vi "Corners to Rectangle Tim's version.vi"(10 "Rectangle Descriptor":T1) -> (2 "output cluster":T3={"diameter points"={"first point"={"x"=0.0, "y"=0.0}, "projected point"={"x"=0.0, "y"=0.0}}, "normalized center"={"x"=0.0, "y"=0.0}, "Overall Score"=0.0, "Distance (ft)"=0.0, "Offset Angle"=0.0, "Tag corner points"=[], "Tag Center"={"X"=0.0, "Y"=0.0}, "Tag Yaw"=0.0, "Tag Pitch"=0.0, "Target Roll (deg)"=0.0, "AprilTag Number"=68} {"Tag Center"."Y" format="%0.2f"; "Tag Center"."X" format="%0.2f"})   [LabVIEW 2023]
uses:
  AprilTag Target Fields.ctl
panel:
  in  "tag info":T2={"tag ID"=0, "Center"={"X"=0.0, "Y"=0.0}, "homography matrix"=[], "decision margin"=0.0, "Hamming Dist"=0, "corner points"=[], "Tag Family"="36h11"}
  # "Bottom Left"
  # "Bottom Right"
  # "Top Right"
  # "Top Left"
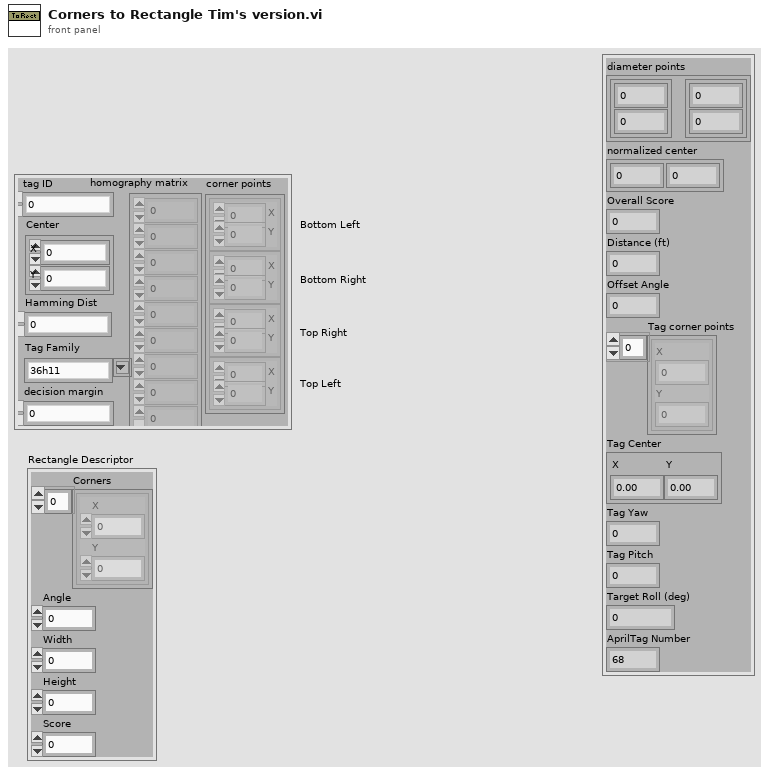
[diagram p1: front panel]
types:
  T1 = cluster{"Corners":cluster{"X":sgl, "Y":sgl}[], "Angle":dbl, "Width":dbl, "Height":dbl, "Score":dbl}
  T2 = cluster{"tag ID":i32, "Center":cluster{"X":dbl, "Y":dbl}, "homography matrix":dbl[], "decision margin":dbl, "Hamming Dist":i32, "corner points":cluster{"X":dbl, "Y":dbl}[], "Tag Family":string}
  T3 = typedef "AprilTag Target Fields.ctl" = cluster{"diameter points":cluster{"first point":cluster{"x":dbl, "y":dbl}, "projected point":cluster{"x":dbl, "y":dbl}}, "normalized center":cluster{"x":dbl, "y":dbl}, "Overall Score":dbl, "Distance (ft)":dbl, "Offset Angle":dbl, "Tag corner points":cluster{"X":dbl, "Y":dbl}[], "Tag Center":cluster{"X":dbl, "Y":dbl}, "Tag Yaw":dbl, "Tag Pitch":dbl, "Target Roll (deg)":dbl, "AprilTag Number":i32}
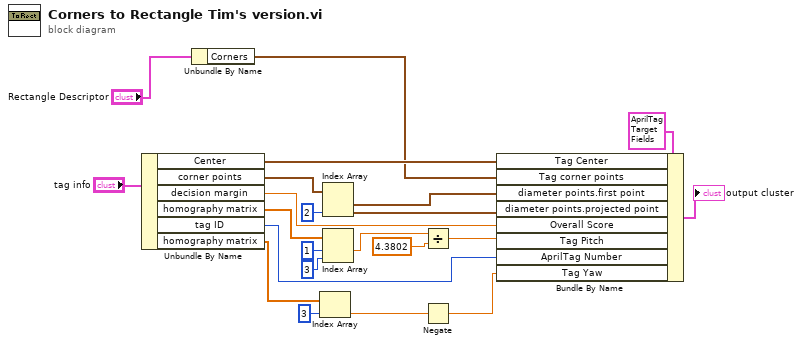
[diagram p0: block diagram]
diagram:
  n1 = Unbundle By Name("tag info") -> ("Center"=w15:cluster{"X":dbl, "Y":dbl}, "corner points"=w14:cluster{"X":dbl, "Y":dbl}[], "decision margin"=w16:dbl, "homography matrix"=w13:dbl[], "tag ID"=w7:i32, "homography matrix"=w6:dbl[])
  n2 = Unbundle By Name("Rectangle Descriptor") -> ("Corners"=w1:cluster{"X":sgl, "Y":sgl}[])
  n3 = Index Array(array=w6, index=3) -> (element=w4:dbl)
  n4 = Index Array(array=w14, index #2=2 ("index")) -> (element #1=w21:cluster{"X":dbl, "Y":dbl}, element #2=w20:cluster{"X":dbl, "Y":dbl})  [unwired: 1 in]
  n5 = Index Array(array=w13, index #1=1 ("index"), index #2=3 ("index")) -> (element #1=w9:dbl)  [unwired: 1 out]
  n6 = Divide(x=w9, y=4.3802) -> (x/y=w8:dbl)
  n7 = Negate(x=w4) -> (-x=w3:dbl)
  n8 = Bundle By Name(cluster=T3 {"diameter points"={"first point"={"x"=0.0, "y"=0.0}, "projected point"={"x"=0.0, "y"=0.0}}, "normalized center"={"x"=0.0, "y"=0.0}, "Overall Score"=0.0, "Distance (ft)"=0.0, "Offset Angle"=0.0, "Tag corner points"=[], "Tag Center"={"X"=0.0, "Y"=0.0}, "Tag Yaw"=0.0, "Tag Pitch"=0.0, "Target Roll (deg)"=0.0, "AprilTag Number"=68} ("results"), "Tag Center"=w15, "Tag corner points"=w1, "diameter points.first point"=w21, "diameter points.projected point"=w20, "Overall Score"=w16, "Tag Pitch"=w8, "AprilTag Number"=w7, "Tag Yaw"=w3) -> (→"output cluster":T3)
